vi "GetCenterPoint.vi"(8 "error in (no error)":errorcluster, 11 "Render Window in":refnum<class "Render Window.lvclass">) -> (0 "error out":errorcluster, 2 "Center Point":cluster{dbl, dbl}, 3 "Render Window out":refnum<class "Render Window.lvclass">)   [LabVIEW 2015, in "Render Window.lvclass"]
uses:
  Render Window.lvclass
  Render Window.lvclass/Render Window.ctl
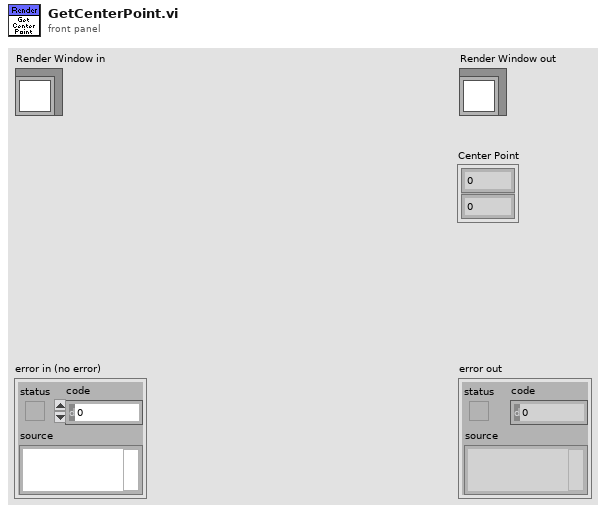
[diagram p1: front panel]
types:
  T1 = typedef "LVRectTypeDef.ctl" = cluster{"Left":i16, "Top":i16, "Right":i16, "Bottom":i16}
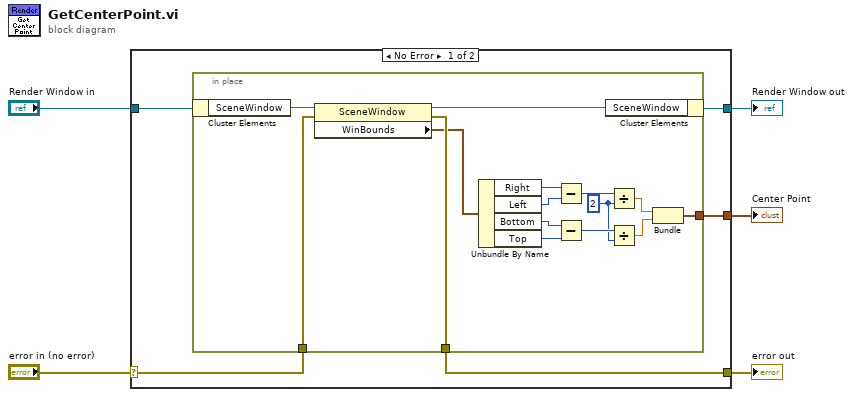
[diagram p0: block diagram]
diagram:
  n1 = case shown="No Error" "error in (no error)" {
    selector: "error in (no error)" -> [w8 w27]
    tunnel: [w7 w27] -> w4
    tunnel: [w9 w26] -> w2
    tunnel: "Render Window in" -> [w10 w26]
    tunnel: [w6 _] -> w1
    frame No Error {
      n2 = in-place {
        in-place-border: w8 -> [w24]
        in-place-border: [w23] -> w7
        in-place-border: [w11] -> w6
        w14 = i16 2 ("y")
        n3 = in-place-cluster #1(w10) -> ("SceneWindow"=w25:refnum<vi>)
        n4 = property class="SceneWindow"(reference=w25, error in=w24) -> (reference out=w22:refnum<vi>, error out=w23:errorcluster, "WinBounds"=w21:T1)
        n5 = Unbundle By Name(w21) -> ("Right"=w20:i16, "Left"=w19:i16, "Bottom"=w18:i16, "Top"=w17:i16)
        n6 = Subtract(x=w20, y=w19) -> (x-y=w16:i16)
        n7 = Subtract(x=w18, y=w17) -> (x-y=w15:i16)
        n8 = in-place-cluster #1("SceneWindow"=w22) -> (w9:refnum<class "Render Window.lvclass">)
        n9 = Divide(x=w16, y=w14) -> (x/y=w13:dbl)
        n10 = Divide(x=w15, y=w14) -> (x/y=w12:dbl)
        n11 = Bundle(w13, w12) -> (w11:cluster{dbl, dbl})  [unwired: 1 in]
      }
    }
    frame Error {
    }
  }
  "error out" <- w4
  "Render Window out" <- w2
  "Center Point" <- w1
